vi "Read_IR_uint32.vi"(4 "node":string, 5 "error in":errorcluster, 8 "Side":T1) -> (0 "error out":errorcluster, 1 "mm/pixel":dbl, 2 "Distance":dbl, 3 "Range":u32)   [LabVIEW 2013]
doc: "Read the IR (either right or left)."
uses:
  ROS/Code/SubVIs/BaxterSide.ctl
  ROS/parsing/primitives/subs/parse_u32_scalar.vi
panel:
  out "Reply":string
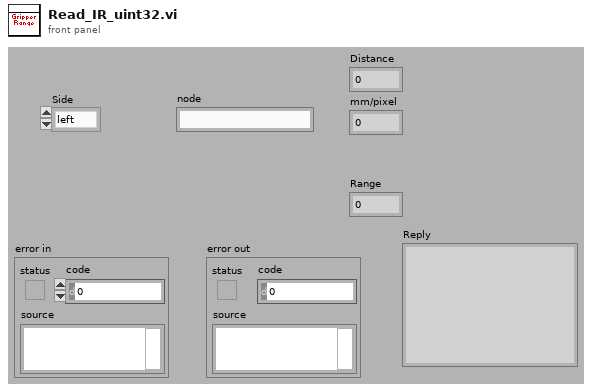
[diagram p1: front panel]
types:
  T1 = typedef "BaxterSide.ctl" = enum16{"left", "right"}
  T2 = enum16{"big-endian, network order", "native, host order", "little-endian"}
  T3 = typedef "_ROSControl.ctl" = cluster{"topic port":u16, "Node":string, "topic":string, "type":string, "node port":u32, "error ":errorcluster, "Direction":T4, "APIs":string[]}
  T4 = typedef "_ROSDirection.ctl" = enum16{"Node", "Publisher", "Subscriber", "Service Client"}
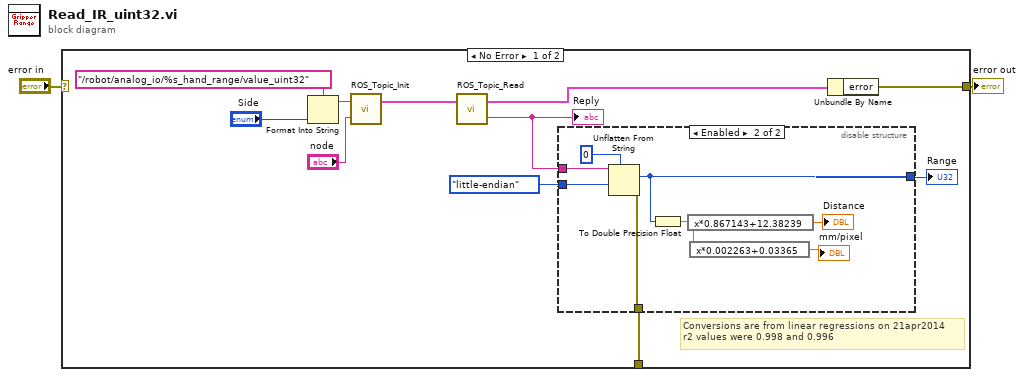
[diagram p0: block diagram]
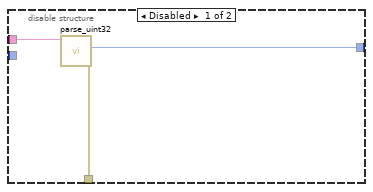
[diagram p2: hidden frame]
diagram:
  n1 = case shown="No Error" "error in" {
    selector: "error in" -> [_ w25]
    tunnel: [w13 w25] -> w2
    tunnel: [w6 _] -> _
    frame No Error {
      # "Conversions are from linear regressions on 21apr2014\nr2 values were 0.998 and 0.996"
      n2 = Format Into String(format string="/robot/analog_io/%s_hand_range/value_uint32" ("topic"), "Side") -> (resulting string=w8:string)  [unwired: 2 in, 1 out]
      n3 = call "ROS_Topic_Init.vi"("node"="node", "topic"=w8) -> ("ROS out"=w11:T3)  [unwired: 1 in]
      n4 = call "ROS_Topic_Read.vi"("ROS in"=w11) -> ("Reply"=w7:string, "ROS out"=w10:T3)  [unwired: 1 in]
      "Reply" <- w7
      n5 = disable-structure shown="Enabled" {
        disable-tunnel: w7 -> [w16 w24]
        disable-tunnel: [w15 w22] -> w6
        disable-tunnel: [w14 w20] -> w4
        disable-tunnel: T2."little-endian" ("byte order (0:big-endian, network order)") -> [_ w21]
        frame Disabled {
          n6 = call-poly "parse_uint32.vi"("msg in"=w16) -> ("error out"=w15:errorcluster, "number"=w14:u32)  [unwired: 4 in, 1 out]
        }
        frame Enabled {
          n7 = Unflatten From String(type=u32 0, binary string=w24, byte order (0:big-endian, network order)=w21) -> (value=w20:u32, error out=w22:errorcluster)  [unwired: 2 in, 1 out]
          n8 = To Double Precision Float(number=w20) -> (double precision float=w19:dbl)
          n9 = expression code="x*0.867143+12.38239"(w19) -> (→"Distance":dbl)
          n10 = expression code="x*0.002263+0.03365"(w19) -> (→"mm/pixel":dbl)
        }
      }
      "Range" <- w4
      n11 = Unbundle By Name(w10) -> ("error"=w13:errorcluster)
    }
    frame Error {
    }
  }
  "error out" <- w2
